vi "create.ReduceSizeLong.vi"(8 "error in (no error)":errorcluster, 11 "ReduceSizeLong.Parameters":T1) -> (0 "error out":errorcluster, 2 "Bytes.out":u8[](array[numeric]) format="%.0x", 3 "ReduceSizeLong":refnum<class "ReduceSizeLong.lvclass">)   [LabVIEW 2020]
uses:
  ReduceSize/ReduceSizeLong.Parameters.ctl
  ReduceSize/ReduceSizeLong.lvclass
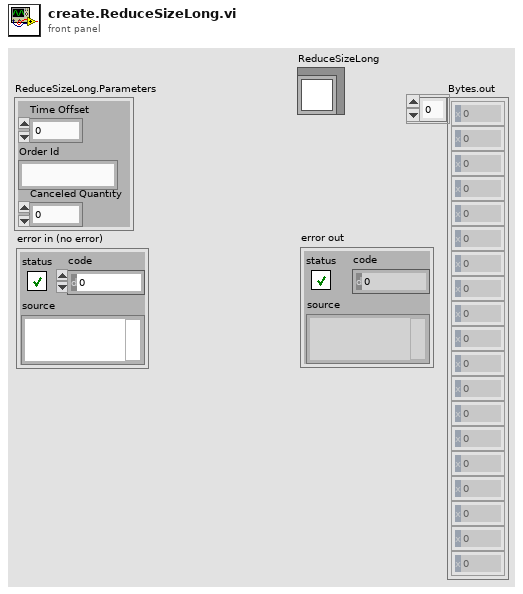
[diagram p1: front panel]
types:
  T1 = typedef "ReduceSizeLong.lvclass/ReduceSizeLong.Parameters.ctl" = cluster{"Time Offset":u32, "Order Id":string, "Canceled Quantity":u32}
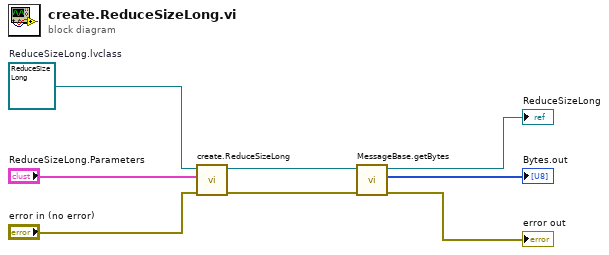
[diagram p0: block diagram]
diagram:
  w8 = refnum<class "ReduceSizeLong.lvclass"> refnum  # ReduceSizeLong.lvclass
  n1 = call-dynamic "create.ReduceSizeLong.vi"("error in (no error)"="error in (no error)", "ReduceSizeLong.Parameters"="ReduceSizeLong.Parameters", "ReduceSizeLong in"=w8) -> ("error out"=w4:errorcluster, "ReduceSizeLong out"=w5:refnum<class "ReduceSizeLong.lvclass">)  [unwired: 7 in]
  n2 = call-dynamic "MessageBase.getBytes.vi"("error in (no error)"=w4, "MessageBase in"=w5) -> ("error out"=→"error out":errorcluster, "Bytes.out"=→"Bytes.out":u8[], "MessageBase out"=→"ReduceSizeLong":refnum<class "ReduceSizeLong.lvclass">)  [unwired: 7 in]
